vi "NE-50X Single Run.vi"() -> ()   [LabVIEW 2020]
doc: "This VI allows to perform a single run pumping mode : the pump run continuously until the user decide to stop, reverse or pause it."
uses:
  <vilib>/Utility/error.llb/DialogType.ctl
panel:
  out "Firmware Version":string
  out "Firmware Version":string
  in  "Secondary Pump Address":i32 format="%0#.0f"
  in  "Master Pump Address":i32 format="%0#.0f"
  out "Tank 2":dbl(slide)
  out "x+y":i32
  out "Tank":dbl(slide)
  in  "PAUSE 2":bool
  in  "Baud Rate (19200)":u32(ring)=19200 items=["19200"=19200, "9600"=9600, "2400"=2400, "1200"=1200, "300"=300]
  in  "VISA resource name":refnum<visa-resource-name>="ASRL1::INSTR"
  in  "PAUSE":bool
  in  "RUN":bool
  in  "STOP":bool
  in  "Audible Alarms":bool=TRUE
  in  "Flow rate\nSee below to enter a right value for flow rate":dbl=0.5 format="%.3f"
  in  "Units":i32(ring) items=["microlitters per minute (µL/min)", "microlitters per hour (µL/hr)", "milliliters per minute (mL/min)", "milliliters per hour (mL/hr)"]
  in  "Initial Direction":u16(ring) items=["Infuse", "Withdraw"]
  in  "Syringe Inside Diameter (19.58 mm)\nIf diameter is upper than 14.00 mm : Volume units are mL\nIf diameter is lower than 14.00 mm : Volume units are µL":dbl=19.58 min=0.1 max=50.0 step=0.01 format="%#_4g"
  out "Status":T1
  out "Volume Dispense":string
  # "Current Status"
  # "Configuration Settings"
  # "Pump System Config"
  # "mm"
  # "RS-232 Setup"
  # "Pump Control"
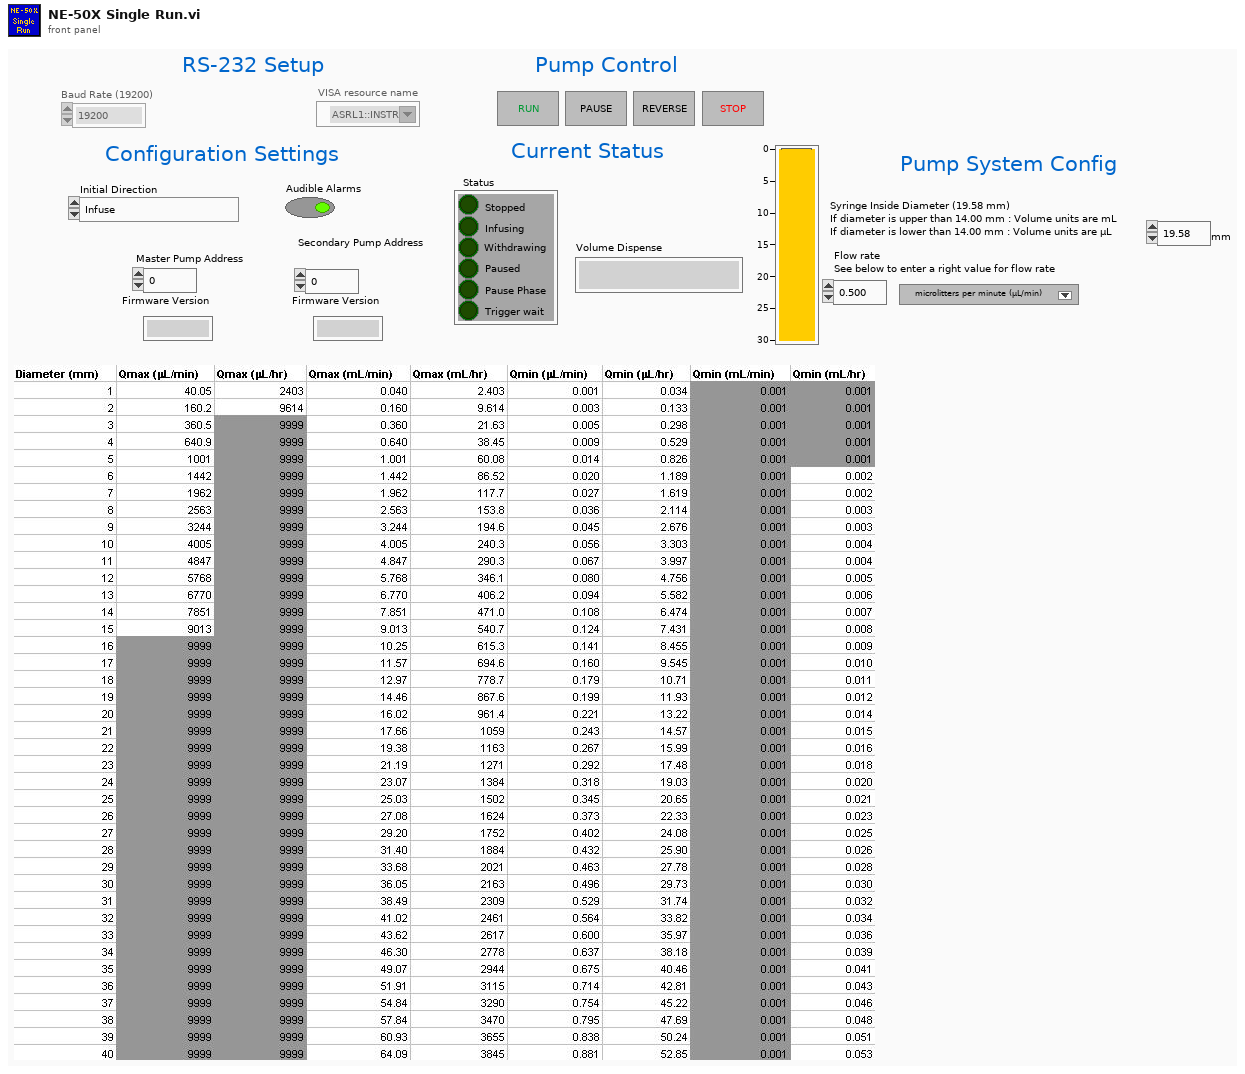
[diagram p1: front panel]
types:
  T1 = cluster{"Stopped":bool, "Infusing":bool, "Withdrawing":bool, "Paused":bool, "Pause Phase":bool, "Trigger wait":bool}
  T2 = typedef "DialogType.ctl" = u16
  T3 = cluster{"0=off\n1=on":u16, "Numbers of beeps\n0=continuously":dbl}
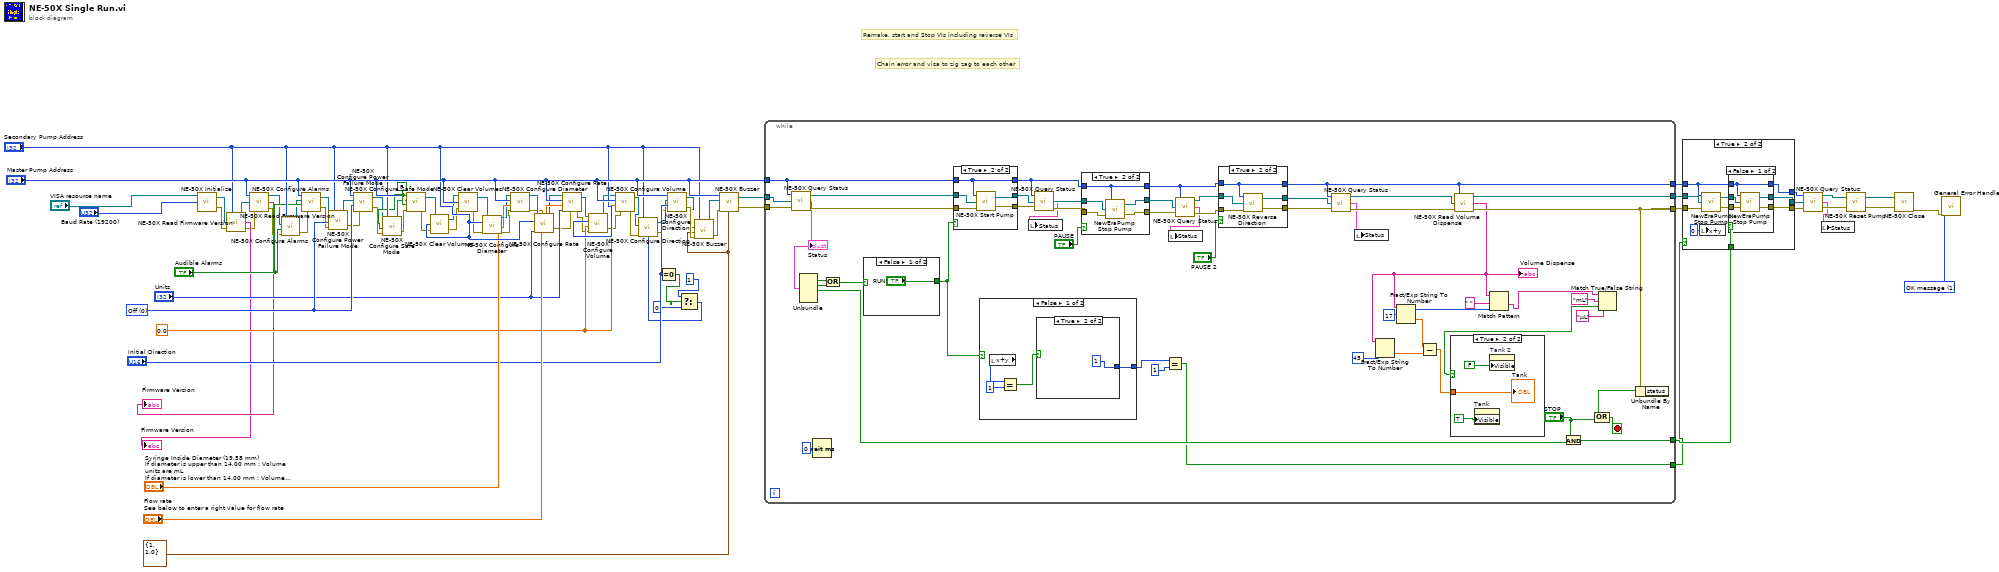
[diagram p0: block diagram]
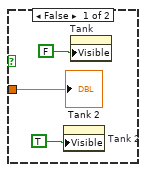
[diagram p4: hidden frame]
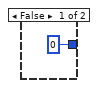
[diagram p5: hidden frame]
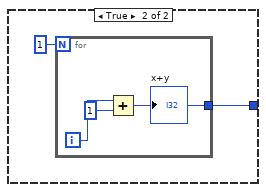
[diagram p6: hidden frame]
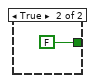
[diagram p7: hidden frame]
diagram:
  w59 = T2 1 items=["no dialog", "OK message", "continue or stop message", "OK message + warnings", "continue/stop + warnings"] ("type of dialog (OK msg:1)")
  w50 = 0.0 ("Volume")
  w54 = FALSE ("0 = Basic")
  w55 = u16 0 items=["Off", "On"] ("0 = Disabled")
  w1 = T3 {"0=off\n1=on"=1, "Numbers of beeps\n0=continuously"=1.0} ("Buzzer")
  # "Chain error and visa to zig zag to each other"
  # "Remake, start and Stop VIs including reverse VIs"
  n1 = call <instrlib>:"NE-50X Initialize.vi"("Baud Rate (19200)"="Baud Rate (19200)", "VISA resource name"="VISA resource name") -> ("error out"=w43:errorcluster, "VISA resource name out"=w40:refnum<visa-resource-name>)  [unwired: 1 in]
  n2 = call <instrlib>:"NE-50X Read Firmware Version.vi"("error in (no error)"=w43, "VISA resource name"=w40, "Address (0)"="Secondary Pump Address") -> ("error out"=w38:errorcluster, "Version"=→"Firmware Version":string, "VISA resource name out"=w39:refnum<visa-resource-name>)
  n3 = call <instrlib>:"NE-50X Read Firmware Version.vi"("error in (no error)"=w38, "VISA resource name"=w39, "Address (0)"="Master Pump Address") -> ("error out"=w36:errorcluster, "Version"=→"Firmware Version":string, "VISA resource name out"=w37:refnum<visa-resource-name>)
  n4 = call <instrlib>:"NE-50X Configure Alarms.vi"("error in (no error)"=w36, "Audible Alarms"="Audible Alarms", "VISA resource name"=w37, "Address (0)"="Secondary Pump Address") -> ("error out"=w35:errorcluster, "VISA resource name out"=w34:refnum<visa-resource-name>)
  n5 = call <instrlib>:"NE-50X Configure Alarms.vi"("error in (no error)"=w35, "Audible Alarms"="Audible Alarms", "VISA resource name"=w34, "Address (0)"="Master Pump Address") -> ("error out"=w33:errorcluster, "VISA resource name out"=w32:refnum<visa-resource-name>)
  n6 = call <instrlib>:"NE-50X Configure Power Failure Mode.vi"("error in (no error)"=w33, "Power Failure Mode"=w55, "VISA resource name"=w32, "Address (0)"="Secondary Pump Address") -> ("error out"=w30:errorcluster, "VISA resource name out"=w31:refnum<visa-resource-name>)
  n7 = call <instrlib>:"NE-50X Configure Power Failure Mode.vi"("error in (no error)"=w30, "Power Failure Mode"=w55, "VISA resource name"=w31, "Address (0)"="Master Pump Address") -> ("error out"=w29:errorcluster, "VISA resource name out"=w26:refnum<visa-resource-name>)
  n8 = call <instrlib>:"NE-50X Configure Safe Mode.vi"("error in (no error)"=w29, "Safe Mode"=w54, "VISA resource name"=w26, "Address (0)"="Secondary Pump Address") -> ("error out"=w28:errorcluster, "VISA resource name out"=w27:refnum<visa-resource-name>)
  n9 = call <instrlib>:"NE-50X Configure Safe Mode.vi"("error in (no error)"=w28, "Safe Mode"=w54, "VISA resource name"=w27, "Address (0)"="Master Pump Address") -> ("error out"=w22:errorcluster, "VISA resource name out"=w25:refnum<visa-resource-name>)
  n10 = call <instrlib>:"NE-50X Clear Volumes.vi"("error in (no error)"=w22, "Address (0)"="Secondary Pump Address", "VISA resource name"=w25) -> ("error out"=w23:errorcluster, "VISA resource name out"=w24:refnum<visa-resource-name>)
  n11 = call <instrlib>:"NE-50X Clear Volumes.vi"("error in (no error)"=w23, "Address (0)"="Master Pump Address", "VISA resource name"=w24) -> ("error out"=w20:errorcluster, "VISA resource name out"=w21:refnum<visa-resource-name>)
  n12 = call <instrlib>:"NE-50X Configure Diameter.vi"("error in (no error)"=w20, "Diameter (19.58 mm)"="Syringe Inside Diameter (19.58 mm)\nIf diameter is upper than 14.00 mm : Volume units are mL\nIf diameter is lower than 14.00 mm : Volume units are µL", "Address (0)"="Secondary Pump Address", "VISA resource name"=w21) -> ("error out"=w18:errorcluster, "VISA resource name out"=w19:refnum<visa-resource-name>)  [unwired: 1 in, 1 out]
  n13 = call <instrlib>:"NE-50X Configure Diameter.vi"("error in (no error)"=w18, "Diameter (19.58 mm)"="Syringe Inside Diameter (19.58 mm)\nIf diameter is upper than 14.00 mm : Volume units are mL\nIf diameter is lower than 14.00 mm : Volume units are µL", "Address (0)"="Master Pump Address", "VISA resource name"=w19) -> ("error out"=w16:errorcluster, "VISA resource name out"=w17:refnum<visa-resource-name>)  [unwired: 1 in, 1 out]
  n14 = call <instrlib>:"NE-50X Configure Rate.vi"("VISA resource name"=w17, "Address (0)"="Secondary Pump Address", "Flow"="Flow rate\nSee below to enter a right value for flow rate", "Units"="Units", "error in (no error)"=w16) -> ("VISA resource name out"=w15:refnum<visa-resource-name>, "error out"=w14:errorcluster)
  n15 = call <instrlib>:"NE-50X Configure Rate.vi"("VISA resource name"=w15, "Address (0)"="Master Pump Address", "Flow"="Flow rate\nSee below to enter a right value for flow rate", "Units"="Units", "error in (no error)"=w14) -> ("VISA resource name out"=w13:refnum<visa-resource-name>, "error out"=w12:errorcluster)
  n16 = call <instrlib>:"NE-50X Configure Volume.vi"("error in (no error)"=w12, "Volume"=w50, "Address (0)"="Secondary Pump Address", "VISA resource name"=w13) -> ("error out"=w10:errorcluster, "VISA resource name out"=w11:refnum<visa-resource-name>)
  n17 = call <instrlib>:"NE-50X Configure Volume.vi"("error in (no error)"=w10, "Volume"=w50, "Address (0)"="Master Pump Address", "VISA resource name"=w11) -> ("error out"=w8:errorcluster, "VISA resource name out"=w9:refnum<visa-resource-name>)
  n18 = Equal To 0?(x="Initial Direction") -> (x = 0?=w48:bool)
  n19 = Select(t=1, s=w48, f=0) -> (s? t:f=w47:i32)
  n20 = call <instrlib>:"NE-50X Configure Direction.vi"("error in (no error)"=w8, "Direction"=w47, "VISA resource name"=w9, "Address (0)"="Secondary Pump Address") -> ("error out"=w6:errorcluster, "VISA resource name out"=w7:refnum<visa-resource-name>)
  n21 = call <instrlib>:"NE-50X Configure Direction.vi"("error in (no error)"=w6, "Direction"="Initial Direction", "VISA resource name"=w7, "Address (0)"="Master Pump Address") -> ("error out"=w5:errorcluster, "VISA resource name out"=w3:refnum<visa-resource-name>)
  n22 = call <instrlib>:"NE-50X Buzzer.vi"("error in (no error)"=w5, "Buzzer"=w1, "VISA resource name"=w3, "Address (0)"="Secondary Pump Address") -> ("error out"=w4:errorcluster, "VISA resource name out"=w2:refnum<visa-resource-name>)
  n23 = call <instrlib>:"NE-50X Buzzer.vi"("error in (no error)"=w4, "Buzzer"=w1, "VISA resource name"=w2, "Address (0)"="Master Pump Address") -> ("error out"=w44:errorcluster, "VISA resource name out"=w69:refnum<visa-resource-name>)
  n24 = while {
    tunnel: w69 -> [w101]
    tunnel: w44 -> [w127]
    tunnel: [w122] -> w67
    tunnel: [w121] -> w68
    tunnel: "Master Pump Address" -> [w100]
    tunnel: [w94] -> w66
    tunnel: [w89] -> w63
    tunnel: [w85] -> w61
    stop <- w128 stop-if-true
    n25 = call <instrlib>:"NE-50X Query Status.vi"("error in (no error)"=w127, "VISA resource name"=w101, "Address (0)"=w100) -> ("error out"=w124:errorcluster, "Status"=w116:T1, "VISA resource name out"=w125:refnum<visa-resource-name>)
    "Status" <- w116
    n26 = Unbundle(w116) -> ("Infusing"=w115:bool, "Withdrawing"=w114:bool, "Paused"=w90:bool)  [unwired: 3 out]
    n27 = Wait (ms)(milliseconds to wait=u32 0) -> ()  [unwired: 1 out]
    n28 = Or(x=w115, y=w114) -> (x .or. y?=w113:bool)
    n29 = case shown="False" w113 {
      tunnel: ["RUN" FALSE ("RUN")] -> w86
      frame False {
      }
      frame True {
      }
    }
    n30 = case shown="True" w86 {
      tunnel: w100 -> [w167 w168]
      tunnel: [w166 w172] -> w93
      tunnel: [w165 w171] -> w112
      tunnel: [w167 w168] -> w99
      tunnel: w125 -> [w166 w169]
      tunnel: w124 -> [w165 w170]
      frame False {
      }
      frame True {
        n31 = call <instrlib>:"NE-50X Start Pump.vi"("error in (no error)"=w170, "VISA resource name"=w169, "Address (0)"=w168) -> ("error out"=w171:errorcluster, "VISA resource name out"=w172:refnum<visa-resource-name>)
      }
    }
    n32 = case shown="False" w86 {
      tunnel: [w136 w142] -> w88
      frame False {
        n33 = local read "x+y"() -> (w139:i32)
        n34 = Equal?(x=w139, y=1) -> (x = y?=w137:bool)
        n35 = case shown="True" w137 {
          tunnel: [0 1] -> w136
          frame False {
          }
          frame True {
          }
        }
      }
      frame True {
        n36 = for {
          N: 1 -> [_]
          tunnel: [w144] -> w142
          i -> [w146]
          n37 = Add(x=w146, y=1) -> (x+y=w144:i32)
          "x+y" <- w144
        }
      }
    }
    n38 = call <instrlib>:"NE-50X Query Status.vi"("error in (no error)"=w112, "VISA resource name"=w93, "Address (0)"=w99) -> ("error out"=w111:errorcluster, "Status"=w104:T1, "VISA resource name out"=w110:refnum<visa-resource-name>)
    n39 = local write "Status"(w104) -> ()
    n40 = case shown="True" "PAUSE" {
      tunnel: w99 -> [w159 w160]
      tunnel: w110 -> [w157 w161]
      tunnel: w111 -> [w158 w164]
      tunnel: [w158 w163] -> w109
      tunnel: [w157 w162] -> w98
      tunnel: [w159 w160] -> w97
      frame False {
      }
      frame True {
        n41 = call <instrlib>:"NewEraPump Stop Pump.vi"("error in (no error)"=w164, "VISA resource name"=w161, "Address (0)"=w160) -> ("error out"=w163:errorcluster, "VISA resource name out"=w162:refnum<visa-resource-name>)
      }
    }
    n42 = Equal?(x=w88, y=1) -> (x = y?=w85:bool)
    n43 = call <instrlib>:"NE-50X Query Status.vi"("error in (no error)"=w109, "VISA resource name"=w98, "Address (0)"=w97) -> ("error out"=w107:errorcluster, "Status"=w103:T1, "VISA resource name out"=w108:refnum<visa-resource-name>)
    n44 = local write "Status"(w103) -> ()
    n45 = case shown="True" "PAUSE 2" {
      tunnel: w108 -> [w151 w152]
      tunnel: w97 -> [w149 w153]
      tunnel: [w151 w156] -> w95
      tunnel: [w150 w155] -> w106
      tunnel: w107 -> [w150 w154]
      tunnel: [w149 w153] -> w94
      frame False {
      }
      frame True {
        n46 = call <instrlib>:"NE-50X Reverse Direction.vi"("error in (no error)"=w154, "VISA resource name"=w152, "Address (0)"=w153) -> ("error out"=w155:errorcluster, "VISA resource name out"=w156:refnum<visa-resource-name>)
      }
    }
    n47 = call <instrlib>:"NE-50X Query Status.vi"("error in (no error)"=w106, "VISA resource name"=w95, "Address (0)"=w94) -> ("error out"=w105:errorcluster, "Status"=w102:T1, "VISA resource name out"=w96:refnum<visa-resource-name>)
    n48 = local write "Status"(w102) -> ()
    n49 = call <instrlib>:"NE-50X Read Volume Dispense.vi"("error in (no error)"=w105, "VISA resource name"=w96, "Address (0)"=w94) -> ("error out"=w121:errorcluster, "Volume Dispense"=w84:string, "VISA resource name out"=w122:refnum<visa-resource-name>)
    "Volume Dispense" <- w84
    n50 = Fract/Exp String To Number(string=w84, offset=45) -> (number=w117:dbl)  [unwired: 2 in, 1 out]
    n51 = Fract/Exp String To Number(string=w84, offset=17) -> (offset past number=w82:i32, number=w118:dbl)  [unwired: 2 in]
    n52 = Subtract(x=w118, y=w117) -> (x-y=w77:dbl)
    n53 = Match Pattern(string=w84, regular expression=" ", offset (0)=w82) -> (after substring=w78:string)  [unwired: 3 out]
    n54 = And(x="STOP", y=w90) -> (x .and. y?=w89:bool)
    n55 = Match True/False String(2:"µL" ("false string"), 3:"mL" ("true string"), 4:w78) -> (0:w79:bool)  [unwired: 1 out]
    n56 = case shown="True" w79 {
      tunnel: w77 -> [w131 w135]
      frame False {
        n57 = property on="Tank 2" class="Slide (strict)"("Visible"=TRUE) -> ()  [unwired: 2 in, 2 out]
        n58 = property on="Tank" class="Slide (strict)"("Visible"=FALSE) -> ()  [unwired: 2 in, 2 out]
        "Tank 2" <- w131
      }
      frame True {
        n59 = property on="Tank" class="Slide (strict)"("Visible"=TRUE) -> ()  [unwired: 2 in, 2 out]
        n60 = property on="Tank 2" class="Slide (strict)"("Visible"=FALSE) -> ()  [unwired: 2 in, 2 out]
        "Tank" <- w135
      }
    }
    n61 = Unbundle By Name(w121) -> ("status"=w92:bool)
    n62 = Compound Arithmetic op=OR(w92, "STOP") -> (w128:bool)
  }
  n63 = case shown="True" w61 {
    tunnel: [w173 w185] -> w73
    tunnel: w68 -> [w173 w184]
    tunnel: w67 -> [w174 w183]
    tunnel: w66 -> [w175 w182]
    tunnel: [w174 w181] -> w65
    tunnel: w63 -> [_ w180]
    tunnel: [w175 w179] -> w62
    frame False {
    }
    frame True {
      n64 = local write "x+y"(0 ("x+y")) -> ()
      n65 = call <instrlib>:"NewEraPump Stop Pump.vi"("error in (no error)"=w184, "VISA resource name"=w183, "Address (0)"=w182) -> ("error out"=w178:errorcluster, "VISA resource name out"=w177:refnum<visa-resource-name>)
      n66 = case shown="False" w180 {
        tunnel: w178 -> [w190 w193]
        tunnel: [w189 w193] -> w185
        tunnel: w182 -> [w186 w191]
        tunnel: [w188 w192] -> w181
        tunnel: w177 -> [w187 w192]
        tunnel: [w186 w191] -> w179
        frame False {
          n67 = call <instrlib>:"NewEraPump Stop Pump.vi"("error in (no error)"=w190, "VISA resource name"=w187, "Address (0)"=w186) -> ("error out"=w189:errorcluster, "VISA resource name out"=w188:refnum<visa-resource-name>)
        }
        frame True {
        }
      }
    }
  }
  n68 = call <instrlib>:"NE-50X Query Status.vi"("error in (no error)"=w73, "VISA resource name"=w65, "Address (0)"=w62) -> ("error out"=w71:errorcluster, "Status"=w70:T1, "VISA resource name out"=w72:refnum<visa-resource-name>)
  n69 = local write "Status"(w70) -> ()
  n70 = call <instrlib>:"NE-50X Reset Pump.vi"("error in (no error)"=w71, "VISA resource name"=w72) -> ("error out"=w64:errorcluster, "VISA resource name out"=w75:refnum<visa-resource-name>)
  n71 = call <instrlib>:"NE-50X Close.vi"("VISA resource name"=w75, "error in (no error)"=w64) -> ("error out"=w60:errorcluster)  [unwired: 13 in]
  n72 = call <vilib>:"General Error Handler.vi"("type of dialog (OK msg:1)"=w59, "error in (no error)"=w60) -> ()  [unwired: 9 in, 5 out]
